vi "SETFLUIDSdll.vi"(8 "error in (no error)":errorcluster, 11 "hFld":string) -> (0 "error out":errorcluster, 1 "ierr":i32, 2 "hFld_Length":i32, 3 "hFld out":string)   [LabVIEW 2015]
doc: "subroutine SETFLUIDSdll(hFld, ierr, hFld_length)\n\nCall the SETUP routine without the need to pass ncomp, hrf, hfmix, or herr, or to declare the length of hfld as\n255 or 10000 bytes long. For a pure fluid, hfld simply contains the name of the fluid file (with a path if needed).\nFor a mixture, it contains the names of the constituents in the mixture separated by a |, a semicolon, or an\nasterisk. To load a predefined mixture, call the SETMIXTURE subroutine (which must return the composition\narray and thus cannot be included here). If it is necessary to set the reference state, call SETUP instead. If ierr\ncomes back non-zero, call the ERRMSG routine to obtain it.\n\nExamples:\ncall SETFLUIDS ('ARGON',ierr) (load argon as a pure fluid)\ncall SETFLUIDS ('FLUIDS/NITROGEN.FLD|FLUIDS/ARGON.FLD|FLUIDS/OXYGEN.FLD|',ierr) (for the air mixture, but giving a path as well)\ncall SETFLUIDS ('AIR.PPF',ierr) (load the air mixture, but read from the pseudo-pure file; properties will be slightly different from the *.mix file since they are different models)\ncall SETFLUIDS ('methane * ethane * propane * butane',ierr)\n\nINPUTS:\nhFld -- String of any character length containing the fluid file names\n\nOUTPUTS:\nierr -- Error flag. 0 = Successful (Values are identical to SETUP; a 109 is returned if the number of fluids in hfld is less than icomp.)\nhFld_length -- length of variable hFld (default: 10000)"
uses:
  REFPROP.dll
panel:
  # "REFPROP-SETFLUIDSdll.vi"
  # "subroutine SETFLUIDSdll(hFld, ierr, hFld_length)"
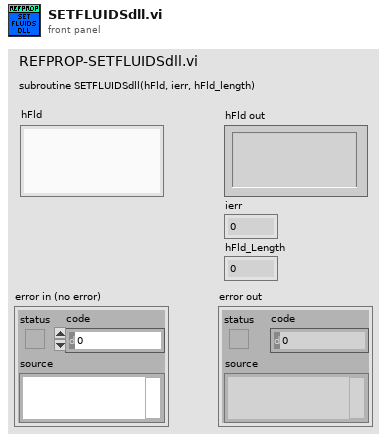
[diagram p1: front panel]
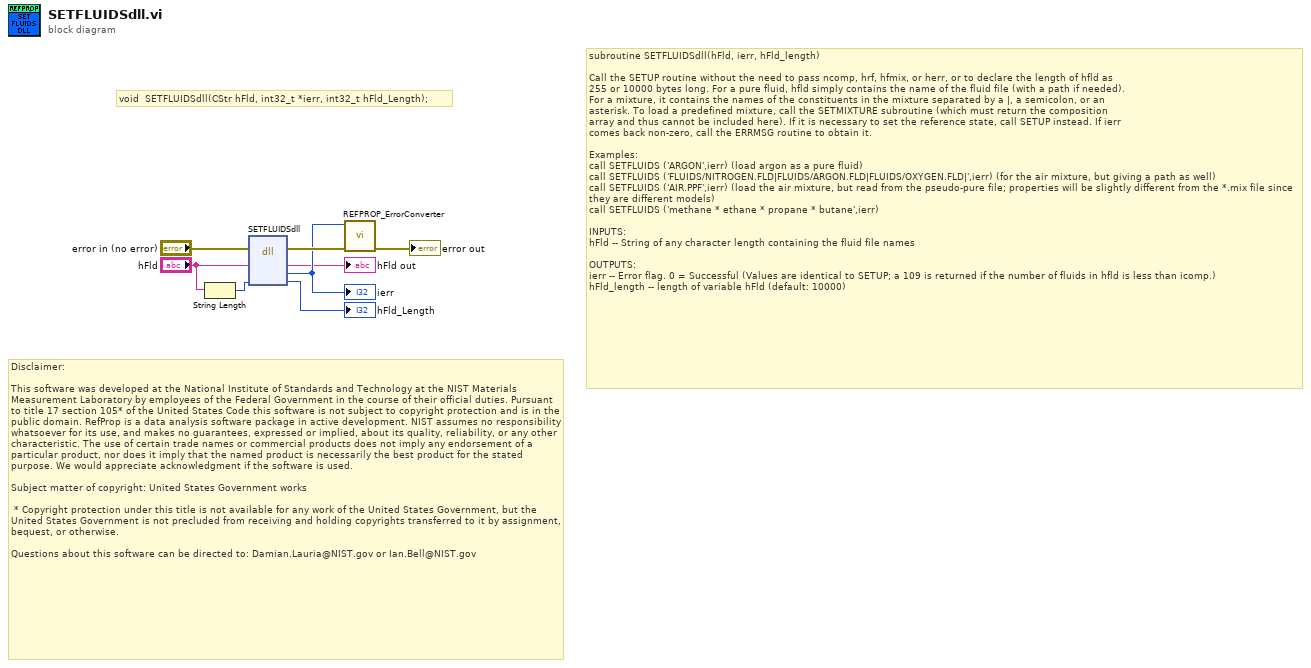
[diagram p0: block diagram]
diagram:
  # "void  SETFLUIDSdll(CStr hFld, int32_t *ierr, int32_t hFld_Length);"
  # "subroutine SETFLUIDSdll(hFld, ierr, hFld_length)\n\nCall the SETUP routine without the need to pass ncomp, hrf, hfmix, or herr, or to declare the length of hfld as\n255 or 10000 bytes long. For a pure fluid, hfld simply contains the name of the fluid file (with a path if needed).\nFor a mixture, it contains the names of the constituents in the mixture separated by a |, a semicolon, or an\nasterisk. To load a predefined mixture, call the SETMIXTURE subroutine (which must return the composition\narray and thus cannot be included here). If it is necessary to set the reference state, call SETUP instead. If ierr\ncomes back non-zero, call the ERRMSG routine to obtain it.\n\nExamples:\ncall SETFLUIDS ('ARGON',ierr) (load argon as a pure fluid)\ncall SETFLUIDS ('FLUIDS/NITROGEN.FLD|FLUIDS/ARGON.FLD|FLUIDS/OXYGEN.FLD|',ierr) (for the air mixture, but giving a path as well)\ncall SETFLUIDS ('AIR.PPF',ierr) (load the air mixture, but read from the pseudo-pure file; properties will be slightly different from the *.mix file since they are different models)\ncall SETFLUIDS ('methane * ethane * propane * butane',ierr)\n\nINPUTS:\nhFld -- String of any character length containing the fluid file names\n\nOUTPUTS:\nierr -- Error flag. 0 = Successful (Values are identical to SETUP; a 109 is returned if the number of fluids in hfld is less than icomp.)\nhFld_length -- length of variable hFld (default: 10000)"
  # "Disclaimer:\n\nThis software was developed at the National Institute of Standards and Technology at the NIST Materials Measurement Laboratory by employees of the Federal Government in the course of their official duties. Pursuant to title 17 section 105* of the United States Code this software is not subject to copyright protection and is in the public domain. RefProp is a data analysis software package in active development. NIST assumes no responsibility whatsoever for its use, and makes no guarantees, expressed or implied, about its quality, reliability, or any other characteristic. The use of certain trade names or commercial products does not imply any endorsement of a particular product, nor does it imply that the named product is necessarily the best product for the stated purpose. We would appreciate acknowledgment if the software is used.\n \nSubject matter of copyright: United States Government works\n  \n * Copyright protection under this title is not available for any work of the United States Government, but the United States Government is not precluded from receiving and holding copyrights transferred to it by assignment, bequest, or otherwise.\n\nQuestions about this software can be directed to: Damian.Lauria@NIST.gov or Ian.Bell@NIST.gov"
  n1 = String Length(string="hFld") -> (length=w2:i32)
  n2 = dll-call lib="C:/Users/lauria/Desktop/REFPROP 10 LabVIEW Wrapper BETA/REFPROP/REFPROP.*" fn="SETFLUIDSdll"(error in="error in (no error)", "hFld"="hFld", "hFld_Length"=w2) -> (error out=w8:errorcluster, "hFld"=→"hFld out":string, "ierr"=w5:i32, "hFld_Length"=→"hFld_Length":i32)  [unwired: 4 in, 1 out]
  "ierr" <- w5
  n3 = call "REFPROP_ErrorConverter.vi"("error in (no error)"=w8, "Error Code"=w5) -> ("error out"=→"error out":errorcluster)  [unwired: 9 in]
